vi "DSF.Shared.Configuration.Framework.Append Suffix.vi"(8 "error in (no error)":errorcluster, 9 "suffix (_0)":string="_0", 10 "string":string, 11 "Framework Configuration in":refnum<class "DSF.Shared.Configuration.Framework.lvclass">) -> (0 "error out":errorcluster, 2 "appended string":string, 3 "Framework Configuration out":refnum<class "DSF.Shared.Configuration.Framework.lvclass">)   [LabVIEW 2017, in "DSF.Shared.lvlib" / "DSF.Shared.Configuration.Framework.lvclass"]
uses:
  DSF.Shared.Configuration.Framework.lvclass
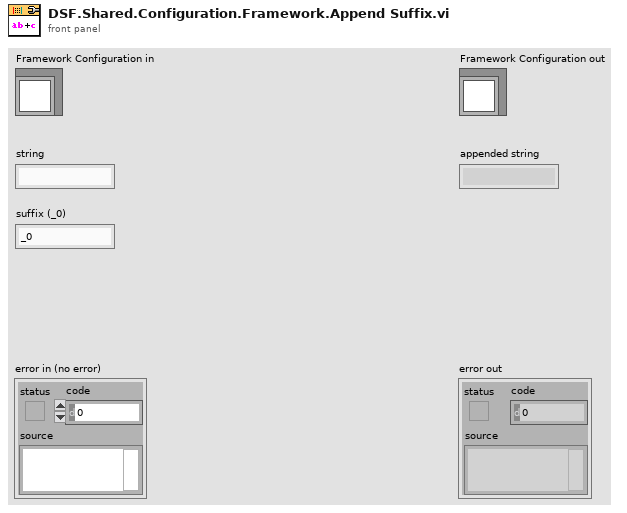
[diagram p1: front panel]
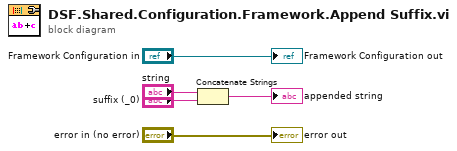
[diagram p0: block diagram]
diagram:
  n1 = Concatenate Strings("string", "suffix (_0)") -> (→"appended string":string)
  "error out" <- "error in (no error)"
  "Framework Configuration out" <- "Framework Configuration in"
